vi "Scroll-Hzoom.vi"(8 "error in (no error)":errorcluster, 9 "Scroll value":i32, 10 "Coords":T1, 11 "Gviewer in":refnum<class "Gviewer.lvclass">) -> (0 "error out":errorcluster, 3 "Gviewer out":refnum<class "Gviewer.lvclass">)   [LabVIEW 2020, in "Sgraph_lib_V1.lvlib" / "Gviewer.lvclass"]
doc: "Andre Koelewijn, 1 may 2021\n\nVertically zoom X-axis using the mouse scroll wheel"
uses:
  Gviewer.lvclass
  <vilib>/Utility/miscctls.llb/LVPoint32TypeDef.ctl
  Gviewer.lvclass/Gviewer.ctl
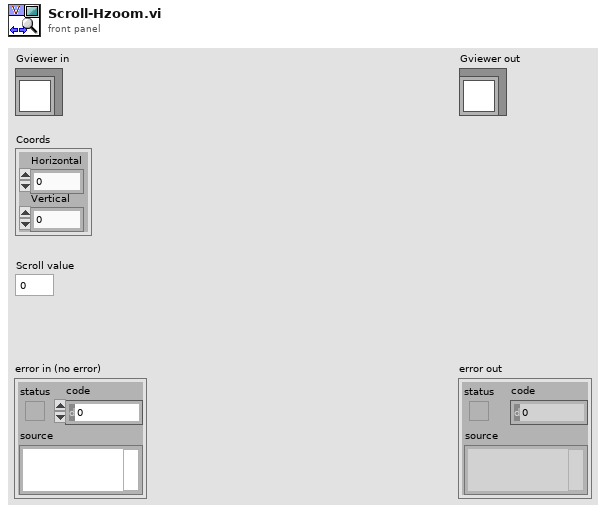
[diagram p1: front panel]
types:
  T1 = typedef "LVPoint32TypeDef.ctl" = cluster{"Horizontal":i32, "Vertical":i32}
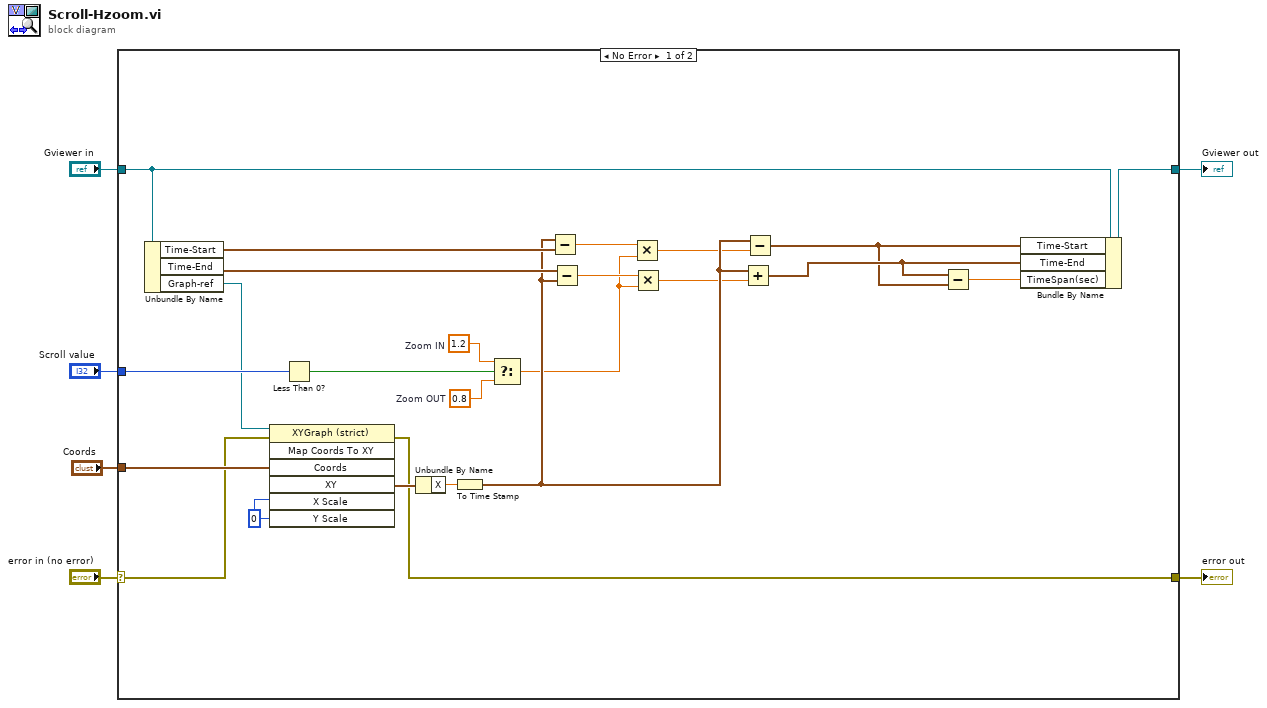
[diagram p0: block diagram]
diagram:
  n1 = case shown="No Error" "error in (no error)" {
    selector: "error in (no error)" -> [w22 w32]
    tunnel: [w21 w32] -> w5
    tunnel: [w29 w31] -> w3
    tunnel: "Gviewer in" -> [w30 w31]
    tunnel: "Scroll value" -> [w28 _]
    tunnel: "Coords" -> [w24 _]
    frame No Error {
      w13 = 0.8  # Zoom OUT
      w14 = 1.2  # Zoom IN
      w26 = 0 ("Y Scale")
      n2 = Unbundle By Name(w30) -> ("Time-Start"=w19:timestamp, "Time-End"=w18:timestamp, "Graph-ref"=w23:refnum<vi>)
      n3 = invoke class="XYGraph (strict)" method="Map Coords To XY"(reference=w23, error in=w22, "Coords"=w24, "X Scale"=w26, "Y Scale"=w26) -> (error out=w21:errorcluster, "XY"=w25:cluster{"X":dbl, "Y":dbl})  [unwired: 2 in, 5 out]
      n4 = Less Than 0?(x=w28) -> (x < 0?=w27:bool)
      n5 = Unbundle By Name(w25) -> ("X"=w20:dbl)
      n6 = To Time Stamp(1:w20) -> (0:w15:timestamp)
      n7 = Select(t=w14, s=w27, f=w13) -> (s? t:f=w12:dbl)
      n8 = Subtract(x=w15, y=w19) -> (x-y=w17:dbl)
      n9 = Subtract(x=w18, y=w15) -> (x-y=w16:dbl)
      n10 = Multiply(x=w17, y=w12) -> (x*y=w11:dbl)
      n11 = Multiply(x=w16, y=w12) -> (x*y=w10:dbl)
      n12 = Add(x=w15, y=w10) -> (x+y=w9:timestamp)
      n13 = Subtract(x=w15, y=w11) -> (x-y=w8:timestamp)
      n14 = Subtract(x=w9, y=w8) -> (x-y=w7:dbl)
      n15 = Bundle By Name(cluster=w30, "Time-Start"=w8, "Time-End"=w9, "TimeSpan(sec)"=w7) -> (w29:refnum<class "Gviewer.lvclass">)
    }
    frame Error {
    }
  }
  "error out" <- w5
  "Gviewer out" <- w3
